vi "StartTimer.vi"(1 "exposure time":u32) -> ()   [LabVIEW 2015]
uses:
  lwlscdll.dll
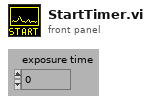
[diagram p1: front panel]
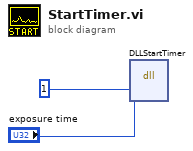
[diagram p0: block diagram]
diagram:
  n1 = dll-call lib="G:/SD/IR-det/lv/2cam/board.vis/lwlscdll.dll" fn="DLLStartTimer"("drv"=u32 1, "exptime"="exposure time") -> ()  [unwired: 6 in, 2 out]
